vi "LINC Read Command (Raw).vi"(8 "error in (no error)":errorcluster, 11 "LINC session":refnum<class "LINC.lvclass">) -> (0 "error out":errorcluster, 1 "cmd data":string, 2 "cmd name":string, 3 "dup LINC session":refnum<class "LINC.lvclass">, 5 "GUID":string, 7 "cmd origin":T1)   [LabVIEW 2018, in "STEPkgDriver_LINC.lvlib" / "LINC.lvclass"]
uses:
  LINC.lvclass
  LINC Global Mode.ctl
  STEPkgDriver_LINC.lvlib
  LINC Global Config Mode.ctl
  LINC Command Origin.ctl
  LINC Command.ctl
  LINC Global Handshake Mode.ctl
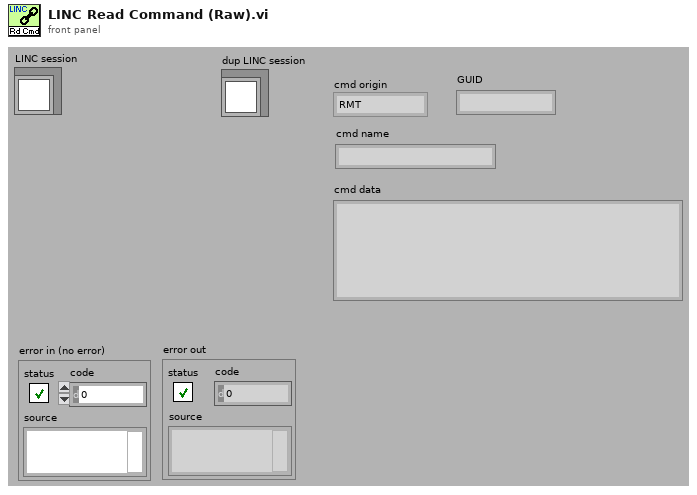
[diagram p1: front panel]
types:
  T1 = typedef "STEPkgDriver_LINC.lvlib/LINC Command Origin.ctl" = enum8{"RMT", "LCL"}
  T2 = typedef "STEPkgDriver_LINC.lvlib/LINC Global Handshake Mode.ctl" = enum16{"INIT", "CLEAR", "ADD_COMMAND", "RMV_COMMAND", "CLR_HANDSHAKE", "SET_HANDSHAKE", "GET_HANDSHAKE"}
  T3 = typedef "STEPkgDriver_LINC.lvlib/LINC Command.ctl" = cluster{"command origin":T1, "command":string, "command data":string}
  T4 = typedef "STEPkgDriver_LINC.lvlib/LINC Global Config Mode.ctl" = enum16{"INIT", "CLEAR", "SET_CMD_CB", "SET_TLM_CB", "SET_CMD_FIELDS", "SET_TLM_FIELDS", "SET_ID", "GET_CONFIG"}
  T5 = typedef "STEPkgDriver_LINC.lvlib/LINC Global Mode.ctl" = enum16{"INIT", "CLEAR", "ADD_PKT_HDR", "ADD_PKT", "GET_PKT_NAMES", "GET_PKT_DESC", "GET_PKT_HDR", "GET_PKT", "SET_PKT", "SET_DATA", "SIM_EN", "SIM_DS"}
  T6 = typedef "STEPkgDriver_LINC.lvlib/LINC Config.ctl" = cluster{"cmd callback":refnum<vi>, "tlm callback":refnum<vi>, "cmd ID bitoffset":i32, "cmd ID bitsize":i32, "cmd IDs":i32[], "tlm ID bitoffset":i32, "tlm ID bitsize":i32, "tlm IDs":i32[], "cmd header fields":i32, "tlm header fields":i32, "tlm header size":i32}
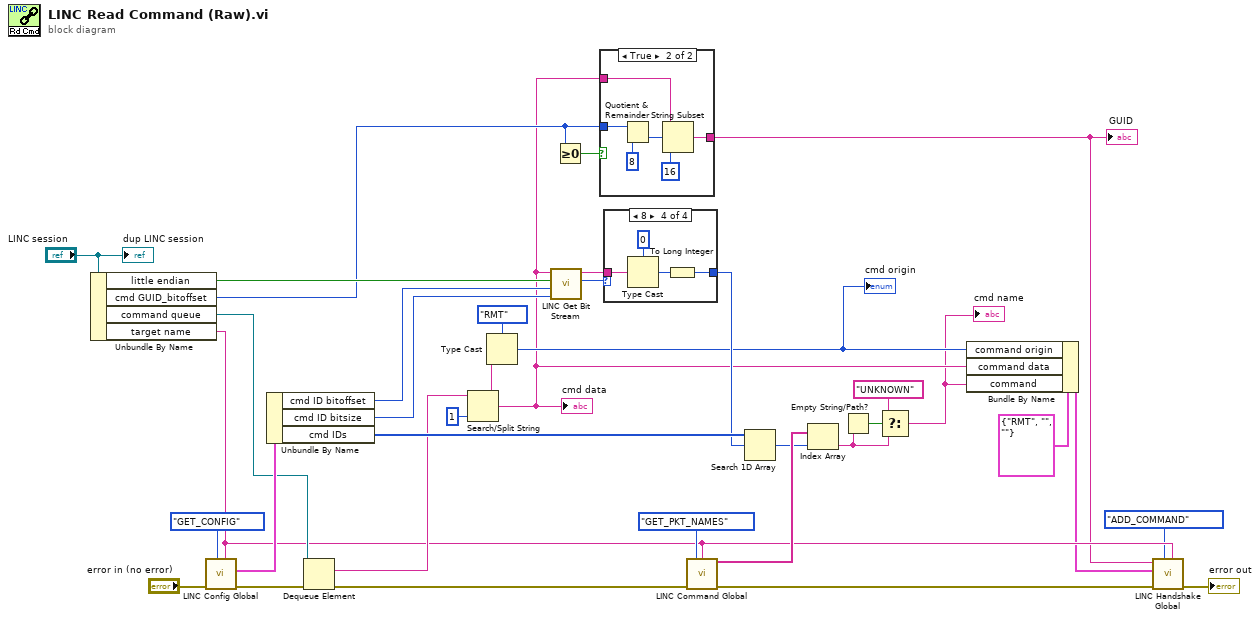
[diagram p0: block diagram]
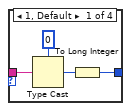
[diagram p3: hidden frame]
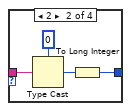
[diagram p4: hidden frame]
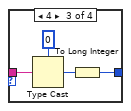
[diagram p5: hidden frame]
diagram:
  n1 = Unbundle By Name("LINC session") -> ("little endian"=w15:bool, "cmd GUID_bitoffset"=w14:i32, "command queue"=w23:refnum<queue>, "target name"=w22:string)
  n2 = call "LINC Config Global.vi"("target name"=w22, "mode"=LINC_Global_Config_Mode."GET_CONFIG", "error in (no error)"="error in (no error)") -> ("error out"=w30:errorcluster, "config out"=w31:T6)  [unwired: 7 in]
  n3 = Unbundle By Name(w31) -> ("cmd ID bitoffset"=w21:i32, "cmd ID bitsize"=w20:i32, "cmd IDs"=w34:i32[])
  n4 = Dequeue Element(queue=w23, error in (no error)=w30) -> (element=w29:string, error out=w26:errorcluster)  [unwired: 1 in, 2 out]
  n5 = Search/Split String(string=w29, offset (0)=1) -> (substring before match=w27:string, match + rest of string=w6:string)  [unwired: 1 in, 1 out]
  "cmd data" <- w6
  n6 = Type Cast(type=LINC_Command_Origin."RMT" ("cmd origin"), x=w27) -> (*(type *) &x=w8:T1)
  "cmd origin" <- w8
  n7 = call "LINC Get Bit Stream.vi"("bit size"=w20, "bit offset"=w21, "little endian"=w15, "data in"=w6) -> ("bytes"=w19:i32, "data out"=w18:string)  [unwired: 6 in]
  n8 = Greater Or Equal To 0?(x=w14) -> (x >= 0?=w13:bool)
  n9 = case shown="True" w13 {
    tunnel: w6 -> [_ w42]
    tunnel: w14 -> [_ w41]
    tunnel: [_ w37] -> w7
    frame False {
    }
    frame True {
      n10 = Quotient & Remainder(x=w41, y=8) -> (floor(x/y)=w39:i32)  [unwired: 1 out]
      n11 = String Subset(string=w42, offset (0)=w39, length (rest)=16 ("length (rest)")) -> (substring=w37:string)
    }
  }
  "GUID" <- w7
  n12 = case shown="8" w19 {
    tunnel: w18 -> [w46 w50 w54 w58]
    tunnel: [w43 w47 w51 w55] -> w17
    frame 1, Default {
      n13 = Type Cast(type=u8 0, x=w46) -> (*(type *) &x=w44:u8)
      n14 = To Long Integer(number=w44) -> (32bit integer=w43:i32)
    }
    frame 2 {
      n15 = Type Cast(type=u16 0, x=w50) -> (*(type *) &x=w48:u16)
      n16 = To Long Integer(number=w48) -> (32bit integer=w47:i32)
    }
    frame 4 {
      n17 = Type Cast(type=u32 0, x=w54) -> (*(type *) &x=w52:u32)
      n18 = To Long Integer(number=w52) -> (32bit integer=w51:i32)
    }
    frame 8 {
      n19 = Type Cast(type=u64 0, x=w58) -> (*(type *) &x=w56:u64)
      n20 = To Long Integer(number=w56) -> (32bit integer=w55:i32)
    }
  }
  n21 = call "LINC Command Global.vi"("mode"=LINC_Global_Mode."GET_PKT_NAMES", "target name"=w22, "error in (no error)"=w26) -> ("values out"=w36:string[], "error out"=w25:errorcluster)  [unwired: 8 in, 3 out]
  n22 = Search 1D Array(1D array=w34, element=w17) -> (index of element=w33:i32)  [unwired: 1 in]
  n23 = Index Array(array=w36, index=w33) -> (element=w3:string)
  n24 = Empty String/Path?(string/path=w3) -> (empty?=w4:bool)
  n25 = Select(t="UNKNOWN", s=w4, f=w3) -> (s? t:f=w1:string)
  "cmd name" <- w1
  n26 = Bundle By Name(cluster=T3 {"command origin"=enum."RMT", "command"="", "command data"=""} ("housekeeping in"), "command origin"=w8, "command data"=w6, "command"=w1) -> (w12:T3)
  n27 = call "LINC Handshake Global.vi"("target name"=w22, "mode"=LINC_Global_Handshake_Mode."ADD_COMMAND", "error in (no error)"=w25, "command in"=w12, "GUID"=w7) -> ("error out"=→"error out":errorcluster)  [unwired: 3 in, 3 out]
  "dup LINC session" <- "LINC session"
